vi "[Challenge] Process N-Channel Array.vi"() -> ()   [LabVIEW 2019]
uses:
  <vilib>/Analysis/4window.llb/windowTd.ctl
  <vilib>/DAQmx/read.llb/DAQmx Read (Analog 1D Wfm NChan NSamp).vi
  <vilib>/DAQmx/create/channels.llb/DAQmx Create Channel (AI-Voltage-Basic).vi
  <vilib>/DAQmx/configure/timing.llb/DAQmx Timing (Sample Clock).vi
  <vilib>/DAQmx/miscellaneous.llb/DAQmx Fill In Error Info.vi
  <vilib>/measure/macond.llb/Scaled Window for N Chan.vi
  <vilib>/measure/maspectr.llb/FFT Power Spectrum and PSD for N Chan.vi
  <resource>/objmgr/daqmx.rc
  <vilib>/measure/NI_MAPro.lvlib
  <vilib>/Analysis/NI_AALPro.lvlib
panel:
  out "Actual Sample Rate (Hz)":dbl
  in  "Desired Sample Rate (Hz)":dbl=2560.0
  in  "Number of Samples":i32=256
  in  "Stop":bool
  out "All Channels":waveform(dbl)[](graph)
  out "Power Spectrum":cluster{"f0":dbl, "df":dbl, "magnitude":dbl[]}[](graph)
  in  "Physical Channels":tag="PCI-6221/ai0, PCI-6221/ai2:3"
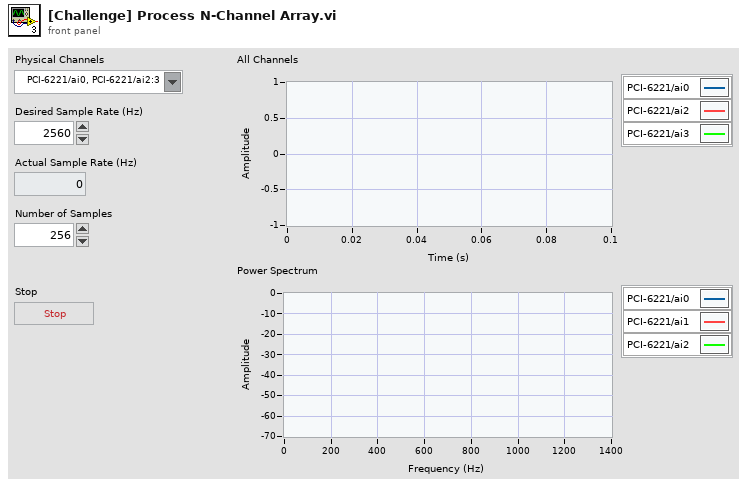
[diagram p1: front panel]
types:
  T1 = typedef "NI_AALPro.lvlib/windowTd.ctl" = u32
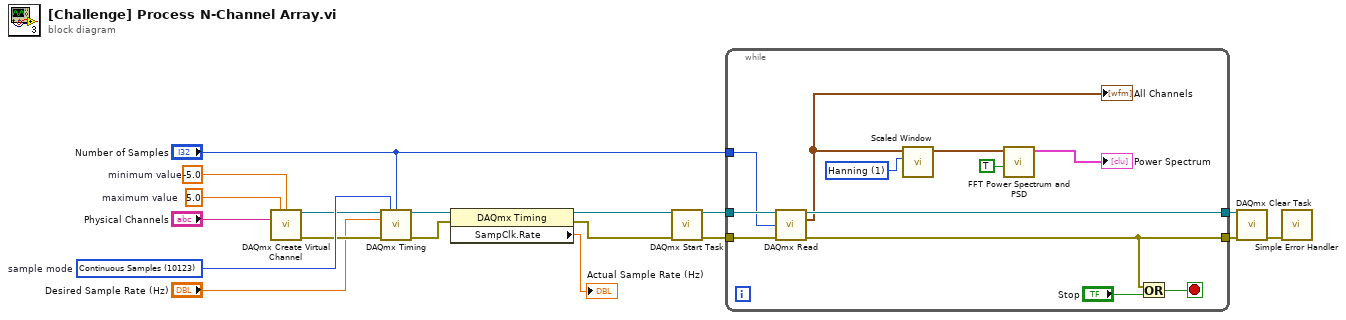
[diagram p0: block diagram]
diagram:
  w13 = 5.0  # maximum value
  w14 = -5.0  # minimum value
  w18 = 10123 items=["Finite Samples"=10178, "Continuous Samples"=10123, "Hardware Timed Single Point"=12522]  # sample mode
  n1 = call-poly <vilib>:"DAQmx Create Virtual Channel.vi"("maximum value"=w13, "minimum value"=w14, "physical channels"="Physical Channels") -> ("task out"=w17:refnum<k21>, "error out"=w16:errorcluster)  [unwired: 11 in]
  n2 = call-poly <vilib>:"DAQmx Timing.vi"("task/channels in"=w17, "sample mode"=w18, "samples per channel"="Number of Samples", "rate"="Desired Sample Rate (Hz)", "error in"=w16) -> ("task out"=w5:refnum<k21>, "error out"=w4:errorcluster)  [unwired: 9 in]
  n3 = property class="DAQmx Timing"(reference=w5, error in=w4) -> (reference out=w3:refnum<k21>, error out=w2:errorcluster, "SampClk.Rate"=→"Actual Sample Rate (Hz)":dbl)
  n4 = call <vilib>:"DAQmx Start Task.vi"("task/channels in"=w3, "error in"=w2) -> ("task out"=w9:refnum<k21>, "error out"=w8:errorcluster)  [unwired: 12 in]
  n5 = while {
    tunnel: [w30] -> w12
    tunnel: [w29] -> w11
    tunnel: w9 -> [w26]
    tunnel: w8 -> [w25]
    tunnel: "Number of Samples" -> [w24]
    stop <- w27 stop-if-true
    w22 = T1 1 items=["Rectangle"=0, "Hanning"=1, "Hamming"=2, "Blackman-Harris"=3, "Exact Blackman"=4, "Blackman"=5, "Flat Top"=6, "4 Term B-Harris "=7, "7 Term B-Harris"=8, "Low Sidelobe"=9, "Blackman Nuttall"=11, "Triangle"=30, "Bartlett-Hanning"=31, "Bohman"=32, "Parzen"=33, "Welch"=34, "Kaiser"=60, "Dolph-Chebyshev"=61, "Gaussian"=62] ("window")
    n6 = call-poly <vilib>:"DAQmx Read.vi"("task/channels in"=w26, "number of samples per channel"=w24, "error in"=w25) -> ("task out"=w30:refnum<k21>, "data"=w23:waveform(dbl)[], "error out"=w29:errorcluster)  [unwired: 10 in]
    "All Channels" <- w23
    n7 = call-poly <vilib>:"Scaled Window.vi"("window"=w22, "signals in"=w23) -> ("signals out"=w21:waveform(dbl)[])  [unwired: 7 in, 2 out]
    n8 = call-poly <vilib>:"FFT Power Spectrum and PSD.vi"("dB On (F)"=TRUE, "time signals"=w21) -> ("Power Spectrum / PSD"=→"Power Spectrum":cluster{"f0":dbl, "df":dbl, "magnitude":dbl[]}[])  [unwired: 6 in, 3 out]
    n9 = Or(x=w29, y="Stop") -> (x .or. y?=w27:bool)
  }
  n10 = call <vilib>:"DAQmx Clear Task.vi"("task in"=w12, "error in"=w11) -> ("error out"=w10:errorcluster)  [unwired: 13 in]
  n11 = call <vilib>:"Simple Error Handler.vi"("error in (no error)"=w10) -> ()  [unwired: 4 in, 5 out]
